vi "FTW-Actor-Log-Error.vi"(0 "FTW Actor Instance":refnum<class "FTW-ActorInstance.lvclass">, 5 "Explanation":string, 11 "Error to Log":errorcluster) -> (4 "FTW Actor Instance out":refnum<class "FTW-ActorInstance.lvclass">, 6 "Exception Occurred?":bool, 8 "Exception":T1, 10 "Serialized Event":string)   [LabVIEW 2013, in "FTW-ActorInstance.lvclass"]
uses:
  FTW-ActorInstance.lvclass
  Error/FTW-ERR-ExceptionType.ctl
  Event/FTW-Event-Level.ctl
panel:
  # "Inputs"
  # "Outputs"
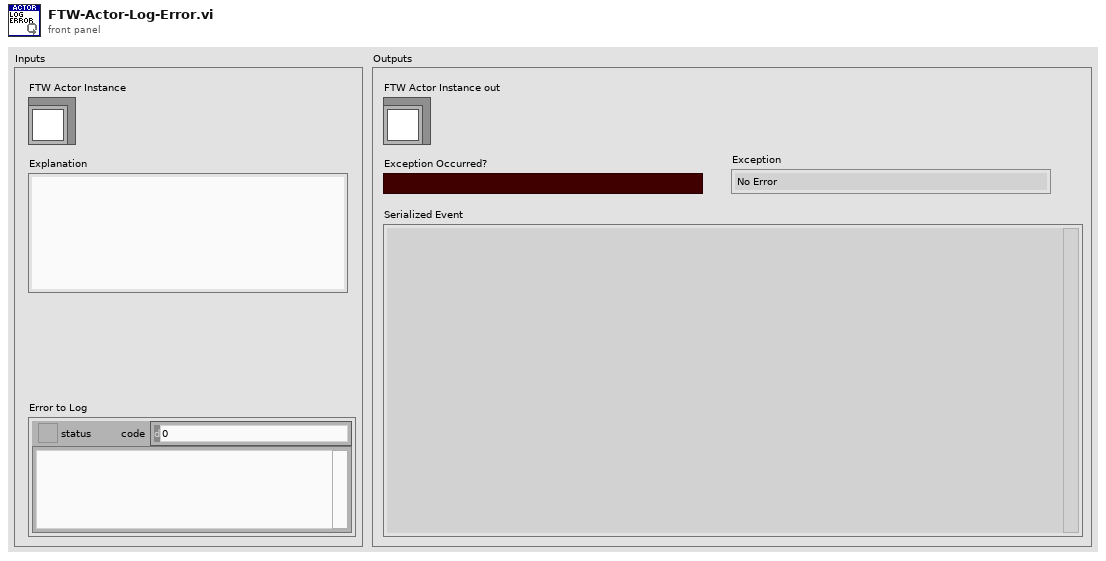
[diagram p1: front panel]
types:
  T1 = typedef "FTW-ERR-ExceptionType.ctl" = enum16{"No Error", "Error", "Warning"}
  T2 = typedef "FTW-Event-Level.ctl" = enum8{"Trace", "Debug", "Information", "Warning", "Error", "Critical"}
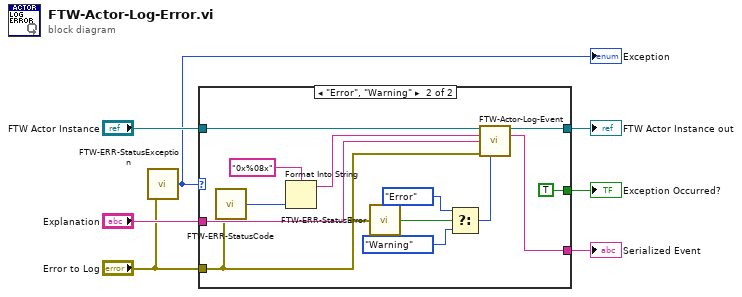
[diagram p0: block diagram]
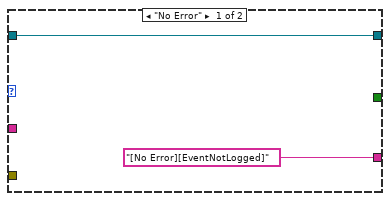
[diagram p2: hidden frame]
diagram:
  n1 = call "FTW-ERR-StatusException.vi"("error to check"="Error to Log") -> ("Exception"=w2:T1)
  "Exception" <- w2
  n2 = case shown="\"Error\", \"Warning\"" w2 {
    tunnel: "Error to Log" -> [_ w12]
    tunnel: "FTW Actor Instance" -> [w9 w21]
    tunnel: [w9 w20] -> w6
    tunnel: [_ TRUE] -> w5
    tunnel: "Explanation" -> [_ w18]
    tunnel: ["[No Error][EventNotLogged]" ("Serialized Event") w17] -> w1
    frame "No Error" {
    }
    frame "Error", "Warning" {
      n3 = call "FTW-ERR-StatusCode.vi"("error to check"=w12) -> ("Code"=w11:i32)
      n4 = Format Into String(format string="0x%08x", w11) -> (resulting string=w19:string)  [unwired: 2 in, 1 out]
      n5 = call "FTW-ERR-StatusError.vi"("error to check"=w12) -> ("Error?"=w15:bool)
      n6 = Select(t=FTW-Event-Level."Error" ("Level"), s=w15, f=FTW-Event-Level."Warning" ("Level")) -> (s? t:f=w14:T2)
      n7 = call-dynamic "FTW-Actor-Log-Event.vi"("FTW Actor Instance"=w21, "Event Type"=w19, "Event Data"=w18, "error in"=w12, "Level"=w14) -> ("FTW Actor Instance out"=w20:refnum<class "FTW-ActorInstance.lvclass">, "Serialized Event"=w17:string)  [unwired: 8 in, 1 out]
    }
  }
  "FTW Actor Instance out" <- w6
  "Exception Occurred?" <- w5
  "Serialized Event" <- w1
